vi "Zstd code to error.vi"(9 "error in":errorcluster, 10 "Error code":i32) -> (1 "error in (no error)":errorcluster)   [LabVIEW 2020, in "lvzstd.lvlib"]
uses:
  lvzstd.lvlib
  <vilib>/ErrorRing/Error Ring.xnode
  <vilib>/Utility/error.llb/Error Cluster From Error Code.vi
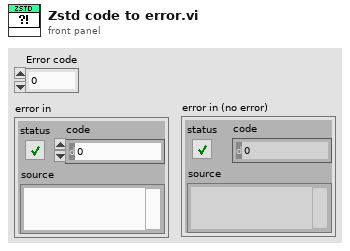
[diagram p1: front panel]
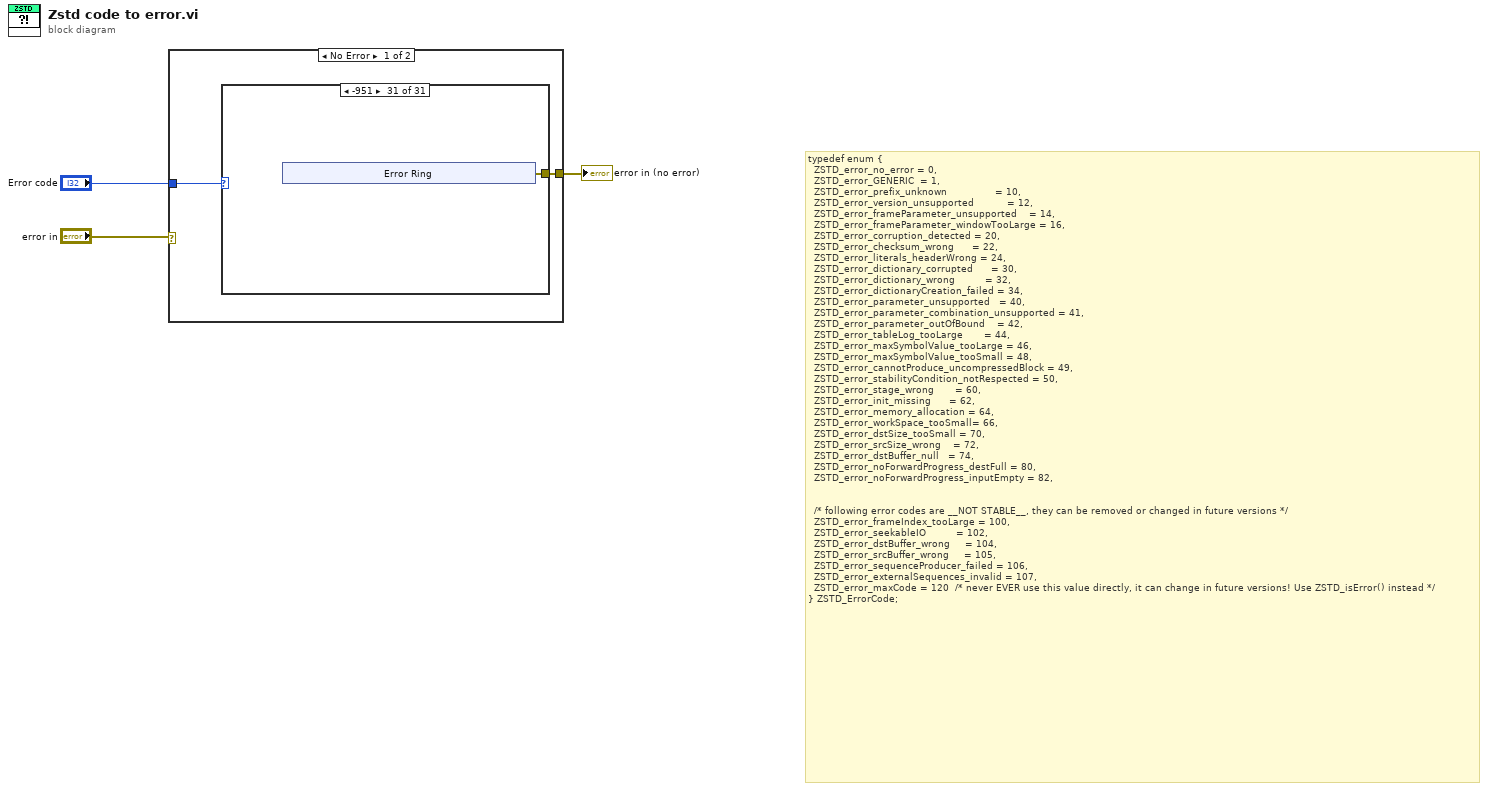
[diagram p0: block diagram]
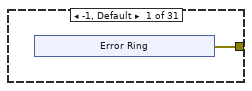
[diagram p2: hidden frame]
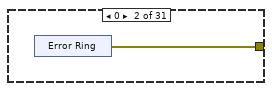
[diagram p3: hidden frame]
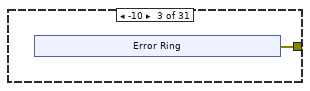
[diagram p4: hidden frame]
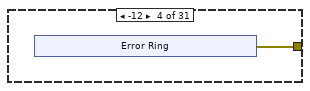
[diagram p5: hidden frame]
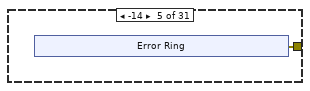
[diagram p6: hidden frame]
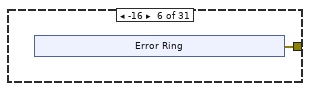
[diagram p7: hidden frame]
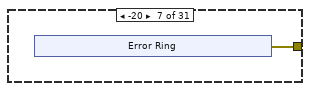
[diagram p8: hidden frame]
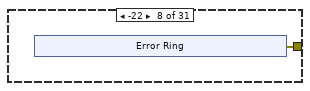
[diagram p9: hidden frame]
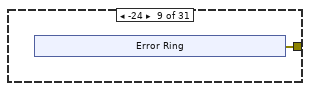
[diagram p10: hidden frame]
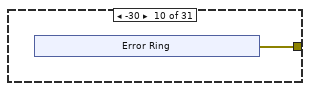
[diagram p11: hidden frame]
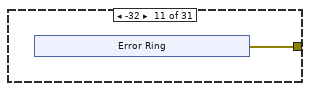
[diagram p12: hidden frame]
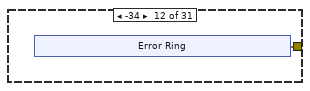
[diagram p13: hidden frame]
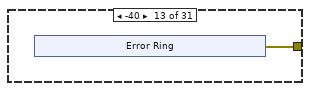
[diagram p14: hidden frame]
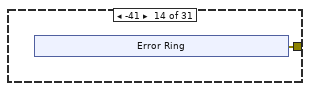
[diagram p15: hidden frame]
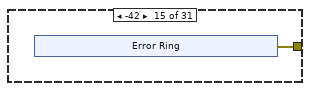
[diagram p16: hidden frame]
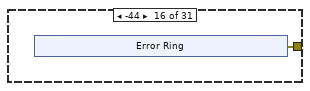
[diagram p17: hidden frame]
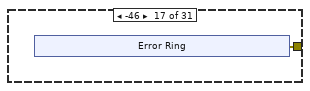
[diagram p18: hidden frame]
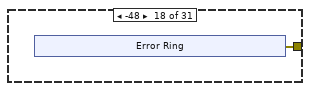
[diagram p19: hidden frame]
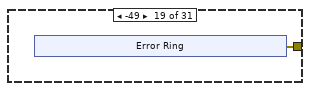
[diagram p20: hidden frame]
diagram:
  # "typedef enum {\n  ZSTD_error_no_error = 0,\n  ZSTD_error_GENERIC  = 1,\n  ZSTD_error_prefix_unknown                = 10,\n  ZSTD_error_version_unsupported           = 12,\n  ZSTD_error_frameParameter_unsupported    = 14,\n  ZSTD_error_frameParameter_windowTooLarge = 16,\n  ZSTD_error_corruption_detected = 20,\n  ZSTD_error_checksum_wrong      = 22,\n  ZSTD_error_literals_headerWrong = 24,\n  ZSTD_error_dictionary_corrupted      = 30,\n  ZSTD_error_dictionary_wrong          = 32,\n  ZSTD_error_dictionaryCreation_failed = 34,\n  ZSTD_error_parameter_unsupported   = 40,\n  ZSTD_error_parameter_combination_unsupported = 41,\n  ZSTD_error_parameter_outOfBound    = 42,\n  ZSTD_error_tableLog_tooLarge       = 44,\n  ZSTD_error_maxSymbolValue_tooLarge = 46,\n  ZSTD_error_maxSymbolValue_tooSmall = 48,\n  ZSTD_error_cannotProduce_uncompressedBlock = 49,\n  ZSTD_error_stabilityCondition_notRespected = 50,\n  ZSTD_error_stage_wrong       = 60,\n  ZSTD_error_init_missing      = 62,\n  ZSTD_error_memory_allocation = 64,\n  ZSTD_error_workSpace_tooSmall= 66,\n  ZSTD_error_dstSize_tooSmall = 70,\n  ZSTD_error_srcSize_wrong    = 72,\n  ZSTD_error_dstBuffer_null   = 74,\n  ZSTD_error_noForwardProgress_destFull = 80,\n  ZSTD_error_noForwardProgress_inputEmpty = 82,\n\n\n  /* following error codes are __NOT STABLE__, they can be removed or changed in future versions */\n  ZSTD_error_frameIndex_tooLarge = 100,\n  ZSTD_error_seekableIO          = 102,\n  ZSTD_error_dstBuffer_wrong     = 104,\n  ZSTD_error_srcBuffer_wrong     = 105,\n  ZSTD_error_sequenceProducer_failed = 106,\n  ZSTD_error_externalSequences_invalid = 107,\n  ZSTD_error_maxCode = 120  /* never EVER use this value directly, it can change in future versions! Use ZSTD_isError() instead */\n} ZSTD_ErrorCode;"
  n1 = case shown="No Error" "error in" {
    selector: "error in" -> [_ w158]
    tunnel: "Error code" -> [w5 _]
    tunnel: [w4 w158] -> w2
    frame No Error {
      n2 = case shown="-951" w5 {
        tunnel: [w6 w11 w13 w18 w23 w28 w33 w38 w43 w48 w53 w58 w63 w68 w73 w78 w83 w88 w93 w98 w103 w108 w113 w118 w123 w128 w133 w138 w143 w148 w153] -> w4
        frame -1, Default {
          n3 = xnode "Error Ring"() -> ("error out"=w6:errorcluster)
        }
        frame 0 {
          n4 = xnode "Error Ring"() -> ("error out"=w11:errorcluster)
        }
        frame -10 {
          n5 = xnode "Error Ring"() -> ("error out"=w13:errorcluster)
        }
        frame -12 {
          n6 = xnode "Error Ring"() -> ("error out"=w18:errorcluster)
        }
        frame -14 {
          n7 = xnode "Error Ring"() -> ("error out"=w23:errorcluster)
        }
        frame -16 {
          n8 = xnode "Error Ring"() -> ("error out"=w28:errorcluster)
        }
        frame -20 {
          n9 = xnode "Error Ring"() -> ("error out"=w33:errorcluster)
        }
        frame -22 {
          n10 = xnode "Error Ring"() -> ("error out"=w38:errorcluster)
        }
        frame -24 {
          n11 = xnode "Error Ring"() -> ("error out"=w43:errorcluster)
        }
        frame -30 {
          n12 = xnode "Error Ring"() -> ("error out"=w48:errorcluster)
        }
        frame -32 {
          n13 = xnode "Error Ring"() -> ("error out"=w53:errorcluster)
        }
        frame -34 {
          n14 = xnode "Error Ring"() -> ("error out"=w58:errorcluster)
        }
        frame -40 {
          n15 = xnode "Error Ring"() -> ("error out"=w63:errorcluster)
        }
        frame -41 {
          n16 = xnode "Error Ring"() -> ("error out"=w68:errorcluster)
        }
        frame -42 {
          n17 = xnode "Error Ring"() -> ("error out"=w73:errorcluster)
        }
        frame -44 {
          n18 = xnode "Error Ring"() -> ("error out"=w78:errorcluster)
        }
        frame -46 {
          n19 = xnode "Error Ring"() -> ("error out"=w83:errorcluster)
        }
        frame -48 {
          n20 = xnode "Error Ring"() -> ("error out"=w88:errorcluster)
        }
        frame -49 {
          n21 = xnode "Error Ring"() -> ("error out"=w93:errorcluster)
        }
        frame -50 {
          n22 = xnode "Error Ring"() -> ("error out"=w98:errorcluster)
        }
        frame -60 {
          n23 = xnode "Error Ring"() -> ("error out"=w103:errorcluster)
        }
        frame -62 {
          n24 = xnode "Error Ring"() -> ("error out"=w108:errorcluster)
        }
        frame -64 {
          n25 = xnode "Error Ring"() -> ("error out"=w113:errorcluster)
        }
        frame -66 {
          n26 = xnode "Error Ring"() -> ("error out"=w118:errorcluster)
        }
        frame -70 {
          n27 = xnode "Error Ring"() -> ("error out"=w123:errorcluster)
        }
        frame -72 {
          n28 = xnode "Error Ring"() -> ("error out"=w128:errorcluster)
        }
        frame -74 {
          n29 = xnode "Error Ring"() -> ("error out"=w133:errorcluster)
        }
        frame -80 {
          n30 = xnode "Error Ring"() -> ("error out"=w138:errorcluster)
        }
        frame -82 {
          n31 = xnode "Error Ring"() -> ("error out"=w143:errorcluster)
        }
        frame -950 {
          n32 = xnode "Error Ring"() -> ("error out"=w148:errorcluster)
        }
        frame -951 {
          n33 = xnode "Error Ring"() -> ("error out"=w153:errorcluster)
        }
      }
    }
    frame Error {
    }
  }
  "error in (no error)" <- w2
